vi "MAC_FPGA.vi"(2 "sin":fxp<+/-,18,1>, 3 "reset":bool, 4 "x":fxp<+/-,24,-10>, 5 "cos":fxp<+/-,18,1>) -> (0 "Imag{}":fxp<+/-,36,0>, 1 "Real{}":fxp<+/-,36,0> format="%.26g")   [LabVIEW 2021]
uses:
  <vilib>/rvi/FXPMathLib/basic elements/FxpIntAccumulator/subVIs/nifxpmath_IntAccumulator_SimConfig.ctl
  <vilib>/rvi/FXPMathLib/basic elements/FxpIntAccumulator/simVIs/DllFxpIntAccumulator_sub.vi
  <vilib>/rvi/FXPMathLib/FxpMul/XNode/nifxpmath_Multiplier.xnode
  <vilib>/rvi/FXPMathLib/basic elements/FxpIntAccumulator/XNode/nifxpmath_IntAccumulator.xnode
  <vilib>/rvi/FXPMathLib/sim/FxpSim.dll
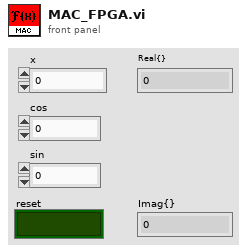
[diagram p1: front panel]
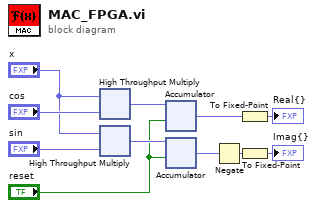
[diagram p0: block diagram]
diagram:
  n1 = xnode ("High Throughput Multiply")("x"="x", "y"="cos") -> ("x*y"=w8:fxp<+/-,42,-9>)
  n2 = xnode ("High Throughput Multiply")("x"="x", "y"="sin") -> ("x*y"=w7:fxp<+/-,42,-9>)
  n3 = xnode "Accumulator"("x"=w8, "load (F)"="reset") -> ("s"=w3:fxp<+/-,51,0>)  [unwired: 3 in, 1 out]
  n4 = xnode "Accumulator"("x"=w7, "load (F)"="reset") -> ("s"=w2:fxp<+/-,51,0>)  [unwired: 3 in, 1 out]
  n5 = Negate(x=w2) -> (-x=w11:fxp<+/-,51,0>)
  n6 = To Fixed-Point(number=w3) -> (fixed-point=→"Real{}":fxp<+/-,36,0>)  [unwired: 1 in]
  n7 = To Fixed-Point(number=w11) -> (fixed-point=→"Imag{}":fxp<+/-,36,0>)  [unwired: 1 in]
